vi "Auto Intake-Elevator-Cangrip.vi"(6 "Intake Wheels (+ is in)":dbl, 7 "Spin Can":enum16{"Spin Left", "Spin Right", "Nothing"}(ring), 8 "Cangrip Open":bool, 9 "Elevator Open":bool, 10 "Intake Open":bool, 11 "Cluster":T12) -> (3 "Output Cluster":T12)   [LabVIEW 2014]
uses:
  <vilib>/Rock Robotics/WPI/Solenoid/WPI_SolenoidDevRef.ctl
  <vilib>/Rock Robotics/WPI/Solenoid/WPI_SolenoidChannel.ctl
  <vilib>/Rock Robotics/WPI/MotorControl/WPI_MotorControlDeviceRef.ctl
  <vilib>/Rock Robotics/WPI/MotorControl/WPI_MotorControlType.ctl
  <vilib>/Rock Robotics/SystemInterfaces/Typedef/FPGA_TypedefDigitalModule.ctl
  <vilib>/Rock Robotics/SystemInterfaces/DIO/FPGA_DIOPWMChannel.ctl
  <vilib>/Rock Robotics/WPI/PWM/WPI_PWMDeadband.ctl
  <vilib>/Rock Robotics/WPI/CAN/Jaguar/SubVIs/WPI_CANJaguar_ControlMode.ctl
  <vilib>/Rock Robotics/WPI/CAN/TalonSRX/WPI_CANTalonSRX_APIControlMode.ctl
  <vilib>/Rock Robotics/WPI/PWM/WPI_PWMTransform_ConPane.ctl
  <vilib>/Rock Robotics/WPI/Solenoid/Deprecated/WPI_SolenoidSetBool.vi
panel:
  in  "Intake Spin Left":bool
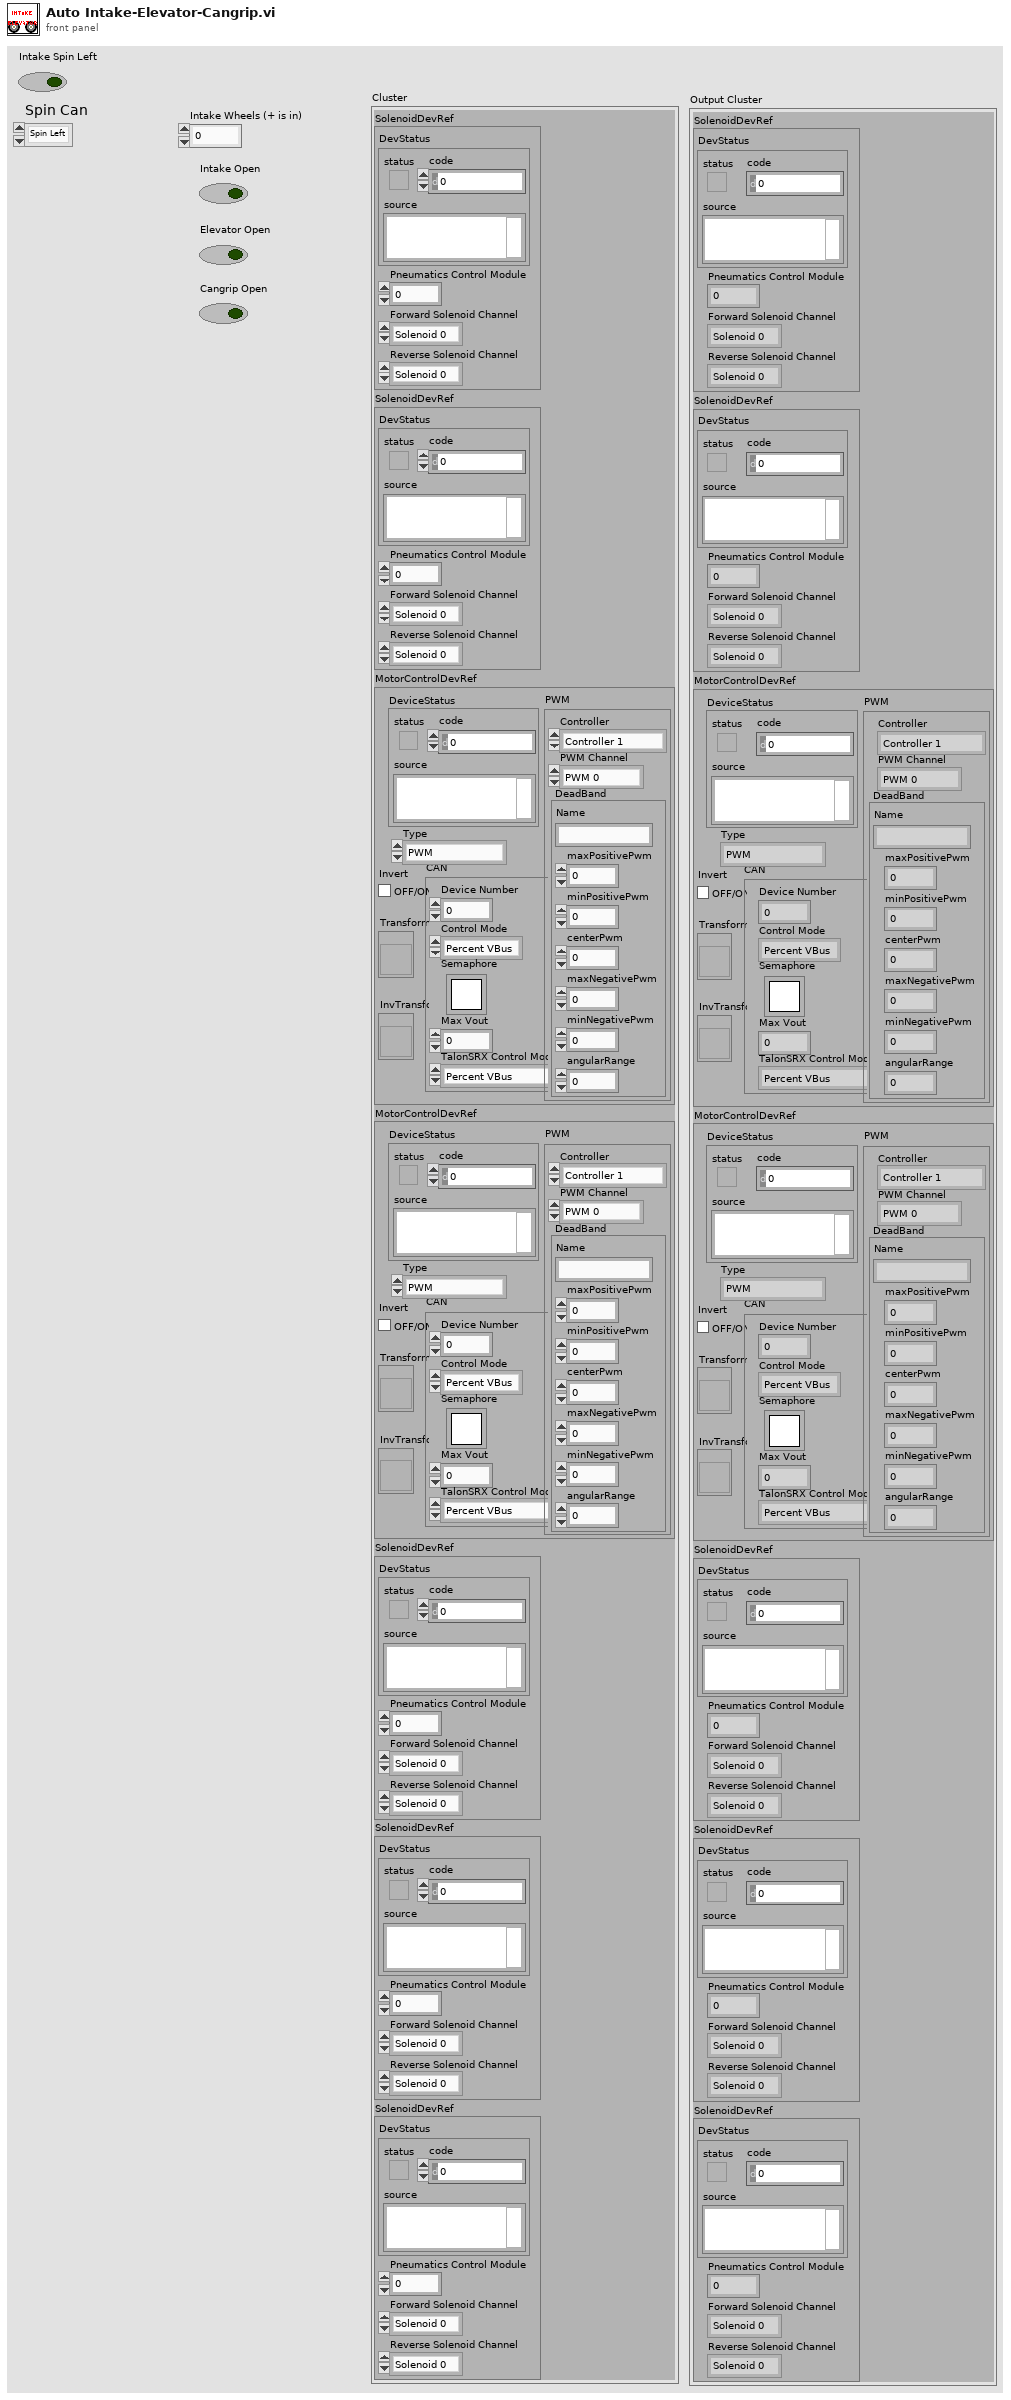
[diagram p1: front panel]
types:
  T1 = typedef "WPI_SolenoidDevRef.ctl" = cluster{"DevStatus":errorcluster, "Pneumatics Control Module":u8, "Forward Solenoid Channel":T2, "Reverse Solenoid Channel":T2}
  T2 = typedef "WPI_SolenoidChannel.ctl" = enum8{"Solenoid 0", "Solenoid 1", "Solenoid 2", "Solenoid 3", "Solenoid 4", "Solenoid 5", "Solenoid 6", "Solenoid 7", "Invalid"}
  T3 = typedef "WPI_MotorControlDeviceRef.ctl" = cluster{"DeviceStatus":errorcluster, "Type":T4, "PWM":cluster{"Controller":T5, "PWM Channel":T6, "DeadBand":T7}, "CAN":cluster{"Device Number":u8, "Control Mode":T8, "Semaphore":T9, "Max Vout":dbl, "TalonSRX Control Mode":T10}, "Invert":bool, "TransformRef":T11, "InvTransformRef":T11}
  T4 = typedef "WPI_MotorControlType.ctl" = enum16{"PWM", "CAN", "CANTalonSRX"}
  T5 = typedef "FPGA_TypedefDigitalModule.ctl" = enum16{"Controller 1"}
  T6 = typedef "FPGA_DIOPWMChannel.ctl" = enum8{"PWM 0", "PWM 1", "PWM 2", "PWM 3", "PWM 4", "PWM 5", "PWM 6", "PWM 7", "PWM 8", "PWM 9", "PWM MXP 0", "PWM MXP 1", "PWM MXP 2", "PWM MXP 3", "PWM MXP 4", "PWM MXP 5", "PWM MXP 6", "PWM MXP 7", "PWM MXP 8", "PWM MXP 9", "Invalid"}
  T7 = typedef "WPI_PWMDeadband.ctl" = cluster{"Name":string, "maxPositivePwm":i32, "minPositivePwm":i32, "centerPwm":i32, "maxNegativePwm":i32, "minNegativePwm":i32, "angularRange":u16}
  T8 = typedef "WPI_CANJaguar_ControlMode.ctl" = enum8{"Percent VBus", "Current", "Speed", "Position", "Voltage"}
  T9 = typedef "Semaphore RefNum" = refnum<k1>
  T10 = typedef "WPI_CANTalonSRX_APIControlMode.ctl" = enum8{"Percent VBus", "Speed", "Position", "Slave", "Unchanged / Invalid"}
  T11 = typedef "WPI_PWMTransform_ConPane.ctl" = refnum<vi>
  T12 = cluster{"SolenoidDevRef":T1, "SolenoidDevRef":T1, "MotorControlDevRef":T3, "MotorControlDevRef":T3, "SolenoidDevRef":T1, "SolenoidDevRef":T1, "SolenoidDevRef":T1}
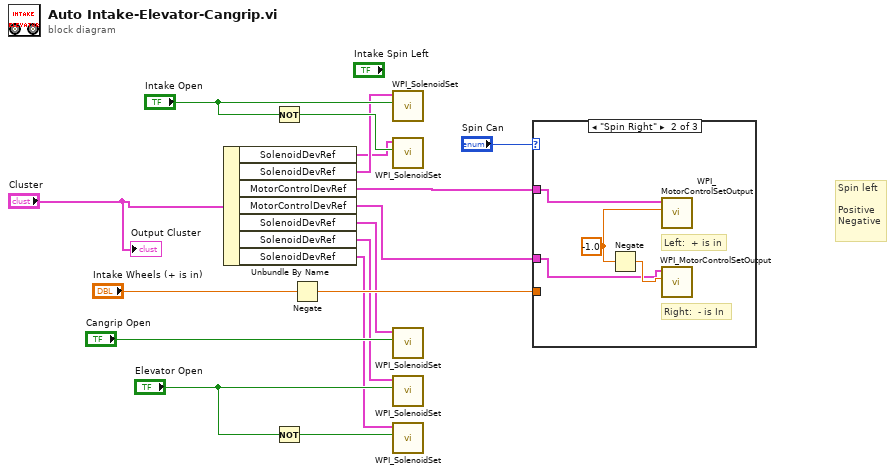
[diagram p0: block diagram]
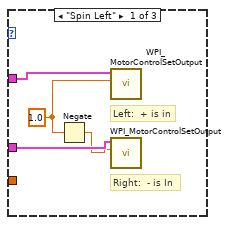
[diagram p2: hidden frame]
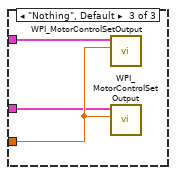
[diagram p3: hidden frame]
diagram:
  # "Spin left\n\nPositive \nNegative"
  n1 = Unbundle By Name("Cluster") -> ("SolenoidDevRef"=w2:T1, "SolenoidDevRef"=w3:T1, "MotorControlDevRef"=w9:T3, "MotorControlDevRef"=w8:T3, "SolenoidDevRef"=w7:T1, "SolenoidDevRef"=w6:T1, "SolenoidDevRef"=w5:T1)
  n2 = Not(x="Intake Open") -> (.not. x?=w16:bool)
  n3 = Not(x="Elevator Open") -> (.not. x?=w15:bool)
  n4 = Negate(x="Intake Wheels (+ is in)") -> (-x=w10:dbl)
  n5 = call-poly <vilib>:"WPI_SolenoidSet.vi"("Value"="Intake Open", "SolenoidDevRef"=w3) -> ()  [unwired: 8 in, 2 out]
  n6 = call-poly <vilib>:"WPI_SolenoidSet.vi"("Value"=w16, "SolenoidDevRef"=w2) -> ()  [unwired: 8 in, 2 out]
  n7 = call-poly <vilib>:"WPI_SolenoidSet.vi"("Value"="Cangrip Open", "SolenoidDevRef"=w7) -> ()  [unwired: 8 in, 2 out]
  n8 = call-poly <vilib>:"WPI_SolenoidSet.vi"("Value"="Elevator Open", "SolenoidDevRef"=w6) -> ()  [unwired: 8 in, 2 out]
  n9 = call-poly <vilib>:"WPI_SolenoidSet.vi"("Value"=w15, "SolenoidDevRef"=w5) -> ()  [unwired: 8 in, 2 out]
  n10 = case shown="\"Spin Right\"" "Spin Can" {
    tunnel: w10 -> [_ _ w27]
    tunnel: w9 -> [w20 w22 w26]
    tunnel: w8 -> [w19 w21 w25]
    frame "Spin Left" {
      w17 = 1.0
      # "Right:  - is In"
      # "Left:  + is in"
      n11 = Negate(x=w17) -> (-x=w18:dbl)
      n12 = call <vilib>:"WPI_MotorControlSetOutput.vi"("Output"=w17, "MotorControlDevRef"=w20) -> ()  [unwired: 7 in, 3 out]
      n13 = call <vilib>:"WPI_MotorControlSetOutput.vi"("Output"=w18, "MotorControlDevRef"=w19) -> ()  [unwired: 7 in, 3 out]
    }
    frame "Spin Right" {
      w23 = -1.0
      # "Right:  - is In"
      # "Left:  + is in"
      n14 = Negate(x=w23) -> (-x=w24:dbl)
      n15 = call <vilib>:"WPI_MotorControlSetOutput.vi"("Output"=w23, "MotorControlDevRef"=w22) -> ()  [unwired: 7 in, 3 out]
      n16 = call <vilib>:"WPI_MotorControlSetOutput.vi"("Output"=w24, "MotorControlDevRef"=w21) -> ()  [unwired: 7 in, 3 out]
    }
    frame "Nothing", Default {
      n17 = call <vilib>:"WPI_MotorControlSetOutput.vi"("Output"=w27, "MotorControlDevRef"=w26) -> ()  [unwired: 7 in, 3 out]
      n18 = call <vilib>:"WPI_MotorControlSetOutput.vi"("Output"=w27, "MotorControlDevRef"=w25) -> ()  [unwired: 7 in, 3 out]
    }
  }
  "Output Cluster" <- "Cluster"
